vi "Set_AcquisitionBuffer.vi"(8 "error in":errorcluster, 9 "PicamAcquisitionBuffer":T1, 11 "device handler in":u64) -> (0 "error out":errorcluster, 3 "device handler out":u64)   [LabVIEW 2019, in "PICam.lvlib"]
doc: "Picam_GetCameraID() returns the ID associates with a specified camera handle."
uses:
  PICam.lvlib
  Picam64.dll   
  Ctrls/PicamAcquisitionBuffer.ctl
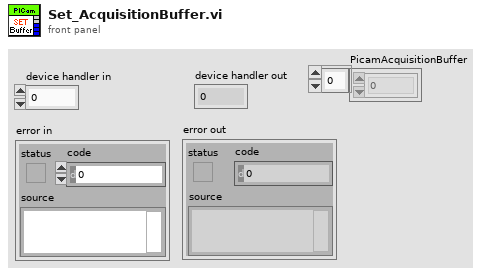
[diagram p1: front panel]
types:
  T1 = typedef "PICam.lvlib/PicamAcquisitionBuffer.ctl" = i8[]
  T2 = cluster{"memory (U32)":u32, "filler (U32)":u32, "memory_size (U64)":u64}
  T3 = cluster{"memory (I64)":i64, "memory_size (I64)":i64}
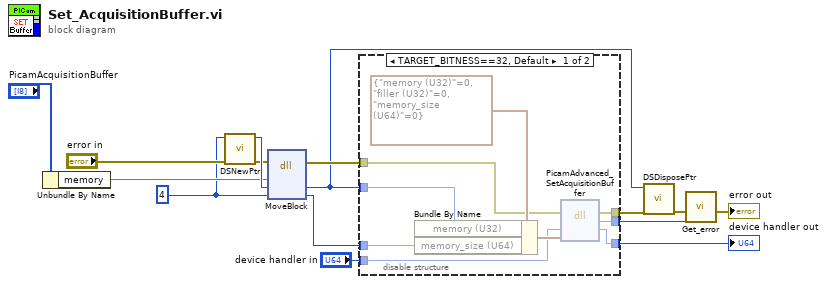
[diagram p0: block diagram]
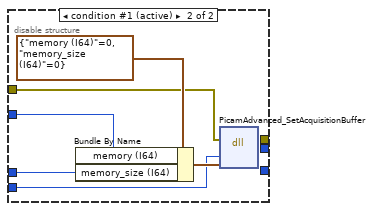
[diagram p2: hidden frame]
diagram:
  w1 = u64 4 ("y")
  n1 = Unbundle By Name("PicamAcquisitionBuffer") -> ("memory"=w2)
  n2 = call <vilib>:"DSNewPtr.vi"("error in (no error)"="error in", "Size"=w1) -> ("error out"=w13:errorcluster, "Pointer"=w14:u64)  [unwired: 8 in]
  n3 = dll-call lib="LabVIEW" fn="MoveBlock"(error in=w13, "src"=w2, "dst"=w14, "size"=w1) -> (error out=w11:errorcluster, "dst"=w9:u64, "size"=w4:u64)  [unwired: 4 in, 1 out]
  n4 = disable-structure shown="TARGET_BITNESS==32, Default" {
    disable-tunnel: w9 -> [w24 w29]
    disable-tunnel: w4 -> [w23 w28]
    disable-tunnel: "device handler in" -> [w20 w27]
    disable-tunnel: w11 -> [w19 w25]
    disable-tunnel: [w18 _] -> w10
    disable-tunnel: [w17 _] -> w7
    disable-tunnel: [w16 _] -> w6
    frame condition #0 {
      n5 = Bundle By Name(cluster=T2 {"memory (U32)"=0, "filler (U32)"=0, "memory_size (U64)"=0}, "memory (U32)"=w24, "memory_size (U64)"=w23) -> (w21:T2)
      n6 = dll-call lib="Picam32.dll" fn="PicamAdvanced_SetAcquisitionBuffer"(error in=w19, "camera_handle"=w20, "PicamAcquisitionBuffer"=w21) -> (error out=w18:errorcluster, "return type"=w17:i32, "camera_handle"=w16:u64)  [unwired: 3 in, 1 out]
    }
    frame condition #1 (active) {
      n7 = Bundle By Name(cluster=T3 {"memory (I64)"=0, "memory_size (I64)"=0}, "memory (I64)"=w29, "memory_size (I64)"=w28) -> (w30:T3)
      n8 = dll-call lib="Picam32.dll" fn="PicamAdvanced_SetAcquisitionBuffer"(error in=w25, "camera_handle"=w27, "PicamAcquisitionBuffer"=w30) -> ()  [unwired: 5 in, 2 out]
    }
  }
  "device handler out" <- w6
  n9 = call <vilib>:"DSDisposePtr.vi"("error in (no error)"=w10, "Pointer"=w9) -> ("error out"=w8:errorcluster)  [unwired: 9 in]
  n10 = call "Get_error.vi"("PICam_Error"=w7, "error in (no error)"=w8) -> ("error out"=→"error out":errorcluster)  [unwired: 9 in]
